vi "SVD_EigSummation.vi"(9 "length":i32, 10 "Start":i32, 11 "Stacked Images":cdb[][][](array[numeric])) -> ()   [LabVIEW 2022 SP3]
panel:
  out "Row Cropped data":dbl[][](graph)
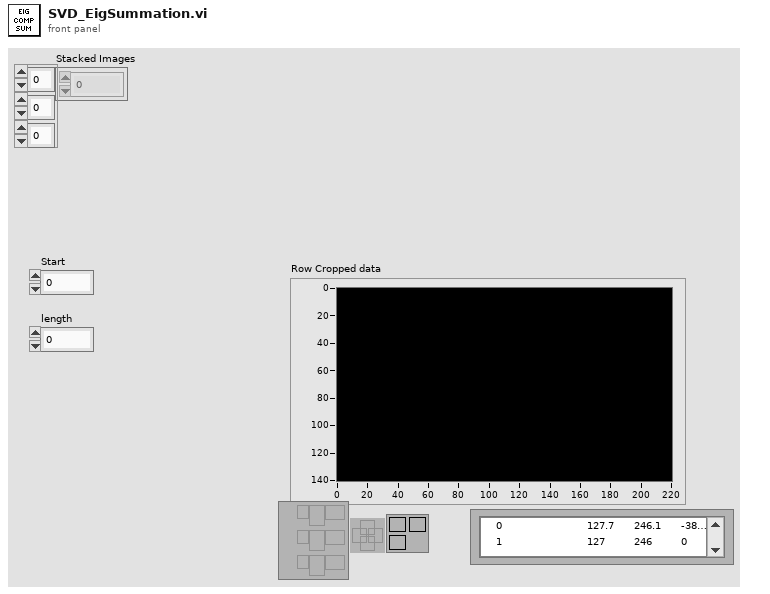
[diagram p1: front panel]
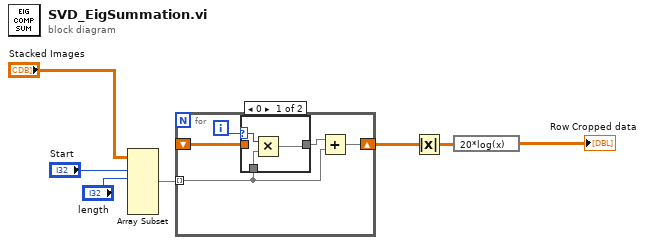
[diagram p0: block diagram]
diagram:
  n1 = Array Subset(array="Stacked Images", index (dim 0)="Start", length (dim 0)="length") -> (w7:cdb[][][])  [unwired: 4 in]
  n2 = for {
    tunnel: w7 -> [w8] mode=indexing
    shift-right: [w12] -> w3
    shift-left: _ -> [w10]
    i -> [w9]
    n3 = case shown="0" w9 {
      selector: w9 -> [w15 _]
      tunnel: [w14 w16] -> w11
      tunnel: w10 -> [_ w16]
      tunnel: w8 -> [w13 _]
      frame 0 {
        n4 = Multiply(x=w15, y=w13) -> (x*y=w14:cdb[][])
      }
      frame 1, Default {
      }
    }
    n5 = Add(x=w11, y=w8) -> (x+y=w12:cdb[][])
  }
  n6 = Absolute Value(x=w3) -> (abs(x)=w4:dbl[][])
  n7 = expression code="20*log(x)"(w4) -> (→"Row Cropped data":dbl[][])
